vi "launcher.vi"   [LabVIEW 2020, in "G-AI Core.lvlib"]
uses:
  G-AI Core/G-AI Core.lvlib
  <vilib>/Delacor/Delacor QMH/Libraries/Module Admin_class/Delacor_lib_QMH_Module Admin.lvclass
  <vilib>/Delacor/Delacor QMH/Libraries/Module Admin_class/Delacor_lib_QMH_Module Admin.lvclass/Delacor_lib_QMH_Module Admin.ctl
  <vilib>/Delacor/Delacor QMH/Libraries/Module Admin_class/Delacor_lib_QMH_Set External Launch.vi
  G-AI Core/Main.vi
panel:
  # "Launcher for G-AI Server. If you see this Frontpanel there was probably an error."
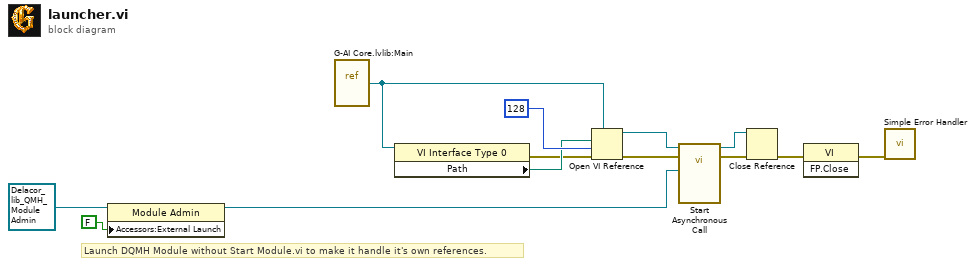
[diagram p0: block diagram]
diagram:
  # "Launch DQMH Module without Start Module.vi to make it handle it's own references."
  n1 = property class="Module Admin"(reference=refnum<class "Delacor_lib_QMH_Module Admin.lvclass"> refnum ("Module Admin"), "Accessors:External Launch"=FALSE ("External Launch")) -> (reference out=w11:refnum<class "Delacor_lib_QMH_Module Admin.lvclass">)  [unwired: 1 in, 1 out]
  n2 = vi-ref "G-AI Core.lvlib:Main.vi"() -> (w8:refnum<vi>)
  n3 = property class="VI Interface Type 0"(reference=w8) -> (error out=w6:errorcluster, "Path"=w7:path)  [unwired: 1 in, 1 out]
  n4 = Open VI Reference(type specifier VI Refnum (for type only)=w8, vi path=w7, options=128, error in (no error)=w6) -> (vi reference=w3:refnum<vi>, error out=w2:errorcluster)  [unwired: 2 in]
  n5 = call-by-ref "Start Asynchronous Call"(reference=w3, error in=w2, "Module Admin"=w11) -> (reference out=w5:refnum<vi>, error out=w4:errorcluster)  [unwired: 11 in]
  n6 = Close Reference(reference=w5, error in (no error)=w4) -> (error out=w1:errorcluster)
  n7 = invoke class="VI" method="FP.Close"(error in=w1) -> (error out=w13:errorcluster)  [unwired: 2 in, 2 out]
  n8 = call <vilib>:"Simple Error Handler.vi"("error in (no error)"=w13) -> ()  [unwired: 4 in, 5 out]
